vi "EncodeNumericValue.vi"(6 "DataLen":i32, 10 "NumericValue":u32, 11 "FrameIn":string) -> (3 "FrameOut":string)   [LabVIEW 2016]
doc: "Concatenate Frame and Numeric Hex String using DataLen. Return concatenated Frame."
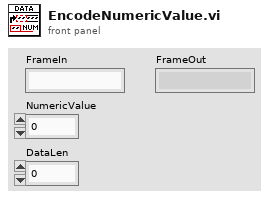
[diagram p1: front panel]
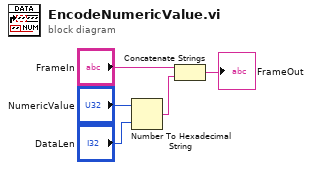
[diagram p0: block diagram]
diagram:
  n1 = Number To Hexadecimal String(1:"DataLen", 2:"NumericValue") -> (0:w5:string)
  n2 = Concatenate Strings("FrameIn", w5) -> (→"FrameOut":string)
